vi "Revision Query.vi"(8 "error in (no error)":errorcluster, 11 "VISA resource name":refnum<visa-resource-name>) -> (0 "error out":errorcluster, 1 "Instr Serial Number":string, 2 "Instr Firmware Revision":string, 3 "VISA resource name out":refnum<visa-resource-name>, 4 "Instr Model Number":string, 5 "Instrument Driver Revision":string, 6 "Option Card Serial Number":string)   [LabVIEW 2015, in "Lake Shore 350.lvlib"]
doc: "Queries the current instrument firmware revision and instrument driver revision.\n\nFor detailed driver information including modification history, refer to the Readme file."
uses:
  Lake Shore 350.lvlib
  Instance           1 22Saved   Revision Query .vi
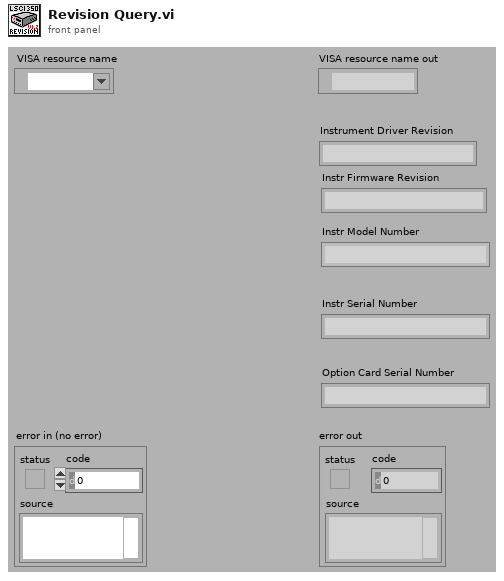
[diagram p1: front panel]
types:
  T1 = cluster{"Major":u16, "Minor":u16, "Fix":u16, "Build":u16}
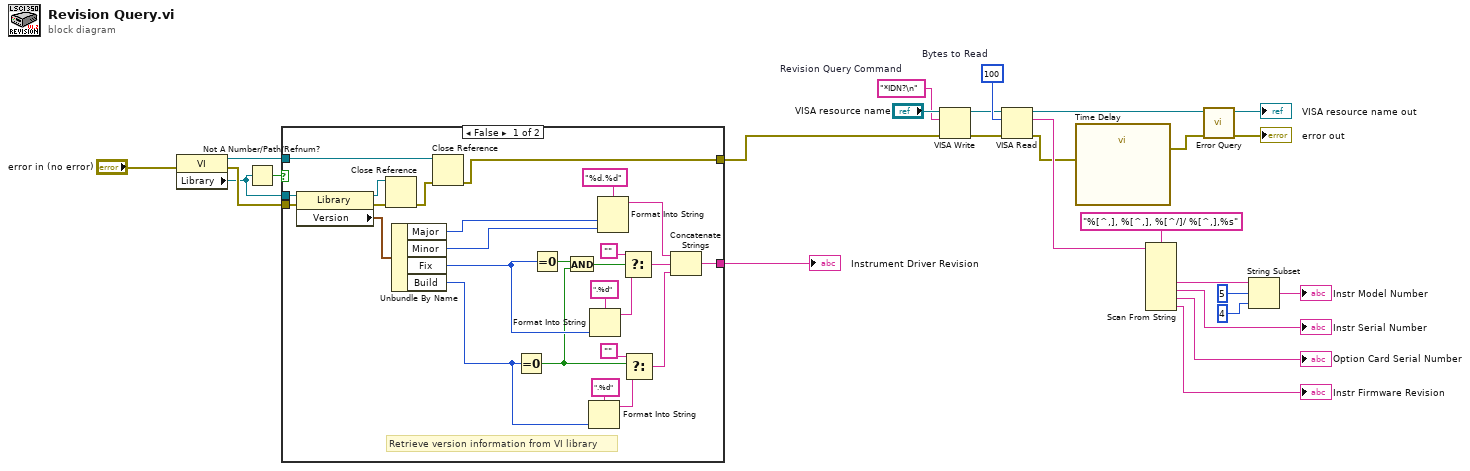
[diagram p0: block diagram]
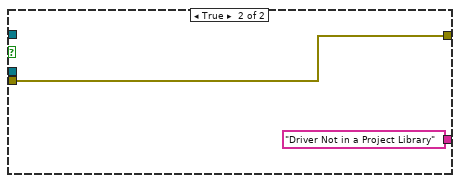
[diagram p2: hidden frame]
diagram:
  w22 = "*IDN?\n"  # Revision Query Command
  w25 = u32 100  # Bytes to Read
  n1 = property on="Property Node" class="VI"(error in="error in (no error)") -> (reference out=w4:refnum<vi>, error out=w3:errorcluster, "Library"=w2:refnum<vi>)  [unwired: 1 in]
  n2 = Not A Number/Path/Refnum?(number/path/refnum=w2) -> (NaN/Path/Refnum?=w1:bool)
  n3 = case shown="False" w1 {
    tunnel: w4 -> [w49 _]
    tunnel: w3 -> [w34 w54]
    tunnel: [w29 w54] -> w17
    tunnel: [w28 "Driver Not in a Project Library"] -> w18
    tunnel: w2 -> [w27 _]
    frame False {
      # "Retrieve version information from VI library"
      n4 = property on="Property Node" class="Library"(reference=w27, error in=w34) -> (reference out=w51:refnum<vi>, error out=w52:errorcluster, "Version"=w48:T1)
      n5 = Close Reference(reference=w51, error in (no error)=w52) -> (error out=w50:errorcluster)
      n6 = Unbundle By Name(w48) -> ("Major"=w37:u16, "Minor"=w36:u16, "Fix"=w33:u16, "Build"=w35:u16)
      n7 = Close Reference(reference=w49, error in (no error)=w50) -> (error out=w29:errorcluster)
      n8 = Equal To 0?(x=w35) -> (x = 0?=w31:bool)
      n9 = Equal To 0?(x=w33) -> (x = 0?=w32:bool)
      n10 = And(x=w32, y=w31) -> (x .and. y?=w30:bool)
      n11 = Format Into String(format string=".%d", w35) -> (resulting string=w41:string)  [unwired: 2 in, 1 out]
      n12 = Format Into String(format string=".%d", w33) -> (resulting string=w45:string)  [unwired: 2 in, 1 out]
      n13 = Format Into String(format string="%d.%d", w37, w36) -> (resulting string=w43:string)  [unwired: 2 in, 1 out]
      n14 = Select(t="" ("Empty String Constant"), s=w30, f=w45) -> (s? t:f=w42:string)
      n15 = Select(t="" ("Empty String Constant"), s=w31, f=w41) -> (s? t:f=w38:string)
      n16 = Concatenate Strings(w43, w42, w38) -> (w28:string)
    }
    frame True {
    }
  }
  "Instrument Driver Revision" <- w18
  n17 = VISA Write(VISA resource name="VISA resource name", write buffer=w22, error in (no error)=w17) -> (VISA resource name out=w24:refnum<visa-resource-name>, error out=w23:errorcluster)  [unwired: 1 out]
  n18 = VISA Read(VISA resource name=w24, byte count=w25, error in (no error)=w23) -> (VISA resource name out=w21:refnum<visa-resource-name>, read buffer=w13:string, error out=w11:errorcluster)  [unwired: 1 out]
  n19 = call "Time Delay"("error in (no error)"=w11) -> ("error out"=w10:errorcluster)  [unwired: 10 in]
  n20 = Scan From String(format string="%[^,], %[^,], %[^/]/ %[^,],%s", input string=w13) -> (output 2=w6:string, output 3=→"Instr Serial Number":string, output 4=→"Option Card Serial Number":string, output 5=→"Instr Firmware Revision":string)  [unwired: 8 in, 3 out]
  n21 = call "Error Query.vi"("error in (no error)"=w10, "VISA resource name"=w21) -> ("error out"=→"error out":errorcluster, "VISA resource name out"=→"VISA resource name out":refnum<visa-resource-name>)  [unwired: 7 in, 1 out]
  n22 = String Subset(string=w6, offset (0)=5, length (rest)=4) -> (substring=→"Instr Model Number":string)
